vi "play_FXP_AFMss_LinearDistEst_singleAxis.vi"() -> ()   [LabVIEW 2017]
uses:
  <vilib>/rvi/interface/nirviMethod/nirviMethod.xnode
  <vilib>/rvi/errors/niLvFpgaMergeErrorWithErrorCode.vi
  <vilib>/rvi/interface/nirviReadWriteControl/nirviReadWriteControl.xnode
  <vilib>/rvi/errors/niLvFpgaAdjustHostInterfaceError.vi
  <vilib>/rvi/interface/nirviOpenFPGA/nirviOpenFPGA.xnode
  <vilib>/userdefined/High Color/nirio_resource_hc.ctl
  <vilib>/FPGAPlugInAG/Dynamic/niLvFpga_Reset_Dynamic.vi
  <vilib>/rvi/interface/Simulation/niFpgaSimulationCallBeginRW.vi
  <vilib>/FPGAPlugInAG/Dynamic/niLvFpga_Run_Dynamic.vi
  <vilib>/rvi/interface/nirviMethod/StockFPGA_InlinedMethodWaitForSingleIRQ.vi
  <vilib>/FPGAPlugInAG/Dynamic/niLvFpga_WaitOnIrq_Dynamic.vi
  <vilib>/FPGAPlugInAG/Dynamic/niLvFpga_AcknowledgeIrq_Dynamic.vi
  <vilib>/rvi/interface/nirviCloseFPGA/nirviCloseFPGA.xnode
  <vilib>/FPGAPlugInAG/Dynamic/niLvFpga_ConfigureFifo_Dynamic.vi
  <vilib>/Utility/error.llb/DialogType.ctl
  <vilib>/Analysis/Matrix/NI_Matrix.lvlib
  fpga_VIs/fpga_subVIs_ssxy/fixed-point-ss/typeDefs/FXPControlParams_distEst.ctl
  <vilib>/FPGAPlugInAG/Dynamic/niLvFpga_WriteFifo_Dynamic.vi
  <vilib>/Analysis/Matrix/Numeric/Conversions/Matrix To Array - RM.vi
  labview/utils_lib/utils.lvlib
  <vilib>/Utility/file.llb/Read Delimited Spreadsheet (DBL).vi
  fpga_interface_lib/fpga_interface.lvlib
  <vilib>/Analysis/Matrix/Numeric/Conversions/Array To Matrix - RA2.vi
  <vilib>/Utility/file.llb/Write To Spreadsheet File (DBL).vi
  fpga_interface_lib/write_FP_data_to_fpga.vi
  <vilib>/Utility/error.llb/Error Cluster From Error Code.vi
  FPGA Bitfiles/afmimagingcontro_FPGATargetSPARTA_FXPAFMssLinearDi_nzyJCj76J+U.lvbitx
  NiFpgaLv.dll
  fpga_interface_lib/acquire_FXP_18-5_FIFO_1.vi
  <vilib>/FPGAPlugInAG/Dynamic/niLvFpga_Close_Dynamic.vi
  <vilib>/FPGAPlugInAG/cRIO-9082/niLvFpga_Open_cRIO-9082.vi
  <vilib>/rvi/interface/common/dynamic/niFpgaDynamicAddResources.vi
  fpga_interface_lib/fpga_interface_types/boolean_indicators.ctl
  <vilib>/Analysis/Matrix/Datatypes/RealMatrix.ctl
panel:
  out "Array":dbl[](array[numeric])
  out "elements left":i32=1
  in  "TF Order":i32
  in  "den":T1
  in  "num":T1
  in  "Tab Control":T2(tab)
  in  "traj_path":path=path "Z:/mpc-journal/step-exps/traj_data.csv"
  in  "TsTicks":i32=1600
  in  "umax":dbl=1.0 format="%#_13g"
  in  "ymax":dbl=4.0 format="%#_13g"
  in  "Iters":i32=25
  in  "SettleTicks":i32=10
  in  "dry_run":bool=TRUE
  in  "control_data_path":path=path "Z:/afm-cs/step-exps/LinControls01.json"
  in  "outputDataPath":path=path "Z:/mpc-journal/step-exps/expOut_multiAxis_tmp.csv"
  out "ControlParams":T3={"umax"=3.0, "Ns_obs/cntrl"=0, "ref_f_VEC"=[0.0, 0.0], "du_max"=0.0, "Nbar"=0.0, "Nhyst"=0, "Nsat"=0, "Ndrift+1"=0}
  in  "ABORT":bool
  out "XY Graph":cluster{dbl[], "2D Data Out":dbl[]}[](graph)
  in  "read_file":bool=TRUE
  in  "All_matrix":T1
  in  "Ns_obs/cntrl":u8=21
  in  "yref":T1
  in  "du_max":dbl=1.0 format="%#_13g"
  out "AllMatrix":dbl[](array[numeric])
  out "ControlMatrices":T4
  out "result_data":T1
  out "boolean  indicators":T5
  out "error out":errorcluster
  out "Empty Elements Remaining":u32
  out "size(s)":i32[](array[numeric])
  out "u_k out":fxp<+/-,32,5>
  out "AllMatHS Length":i32
  # "NOTE: Ns is the number of states in the plant. The number of states in the \nobserver is Ns+1. Thus, for B, L, C, and A, we use NS+1. For K and Xss, we use Ns\nbecause the controller does not operate on the disturbance state, Xd."
  # "yk\nulin\ndu\nu_inv\nIpow\nX"
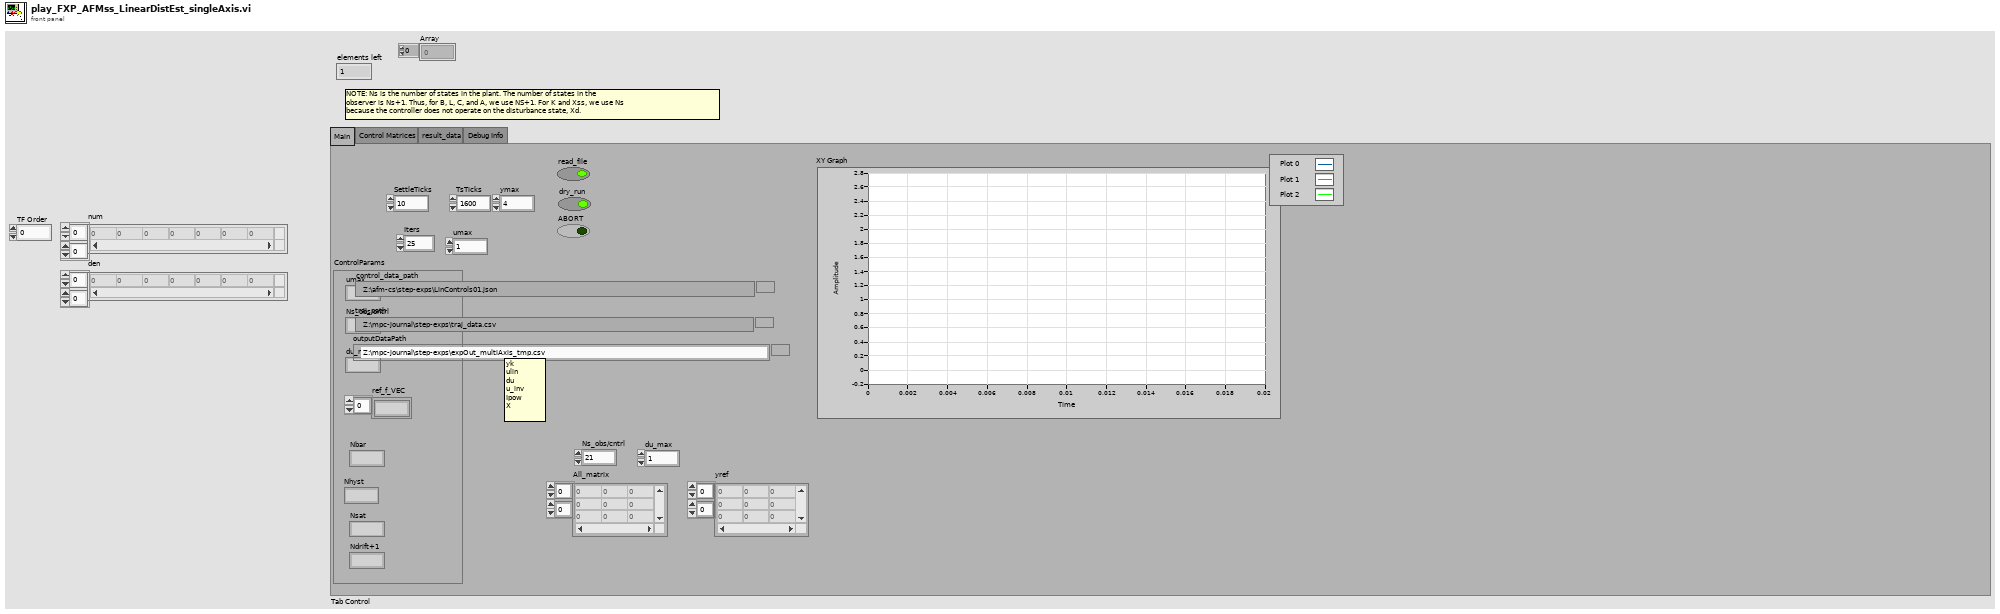
[diagram p1: front panel]
types:
  T1 = typedef "NI_Matrix.lvlib/RealMatrix.ctl" = dbl[][]
  T2 = enum32{"Main", "Control Matrices", "result_data", "Debug Info"}
  T3 = typedef "FXPControlParams_distEst.ctl" = cluster{"umax":fxp<+/-,18,5>, "Ns_obs/cntrl":u8, "ref_f_VEC":fxp<+/-,32,5>[], "du_max":fxp<+/-,18,5>, "Nbar":fxp<+/-,32,5>, "Nhyst":u8, "Nsat":u8, "Ndrift+1":u8}
  T4 = cluster{"Az":fxp<+/-,32,4>[][], "Bz":dbl[][], "Lz":dbl[][], "Kz":dbl[][], "NxNu":dbl[][]}
  T5 = typedef "fpga_interface.lvlib/boolean_indicators.ctl" = cluster{"unstable-z-traj":bool, "input fifo time-out":bool, "logging fifo timeout":bool, "scanning finished":bool, "unstable-x-traj":bool, "unstable-y-traj":bool, "ABORT":bool, "All Measurements Done":bool, "fpga_finished":bool}
  T6 = typedef "nirio_resource_hc.ctl" = tag
  T7 = typedef "ObserverMatrices.ctl" = cluster{"Az":fxp<+/-,32,4>[][], "Bz":dbl[][], "Lz":dbl[][], "Kz":dbl[][], "NxNu":dbl[][]}
  T8 = cluster{"unstable-z-traj":bool, "input fifo time-out":bool, "logging fifo timeout":bool, "scanning finished":bool, "unstable-x-traj":bool, "unstable-y-traj":bool, "ABORT":bool, "All Measurements Done":bool, "fpga_finished":bool}
  T9 = typedef "DialogType.ctl" = u16
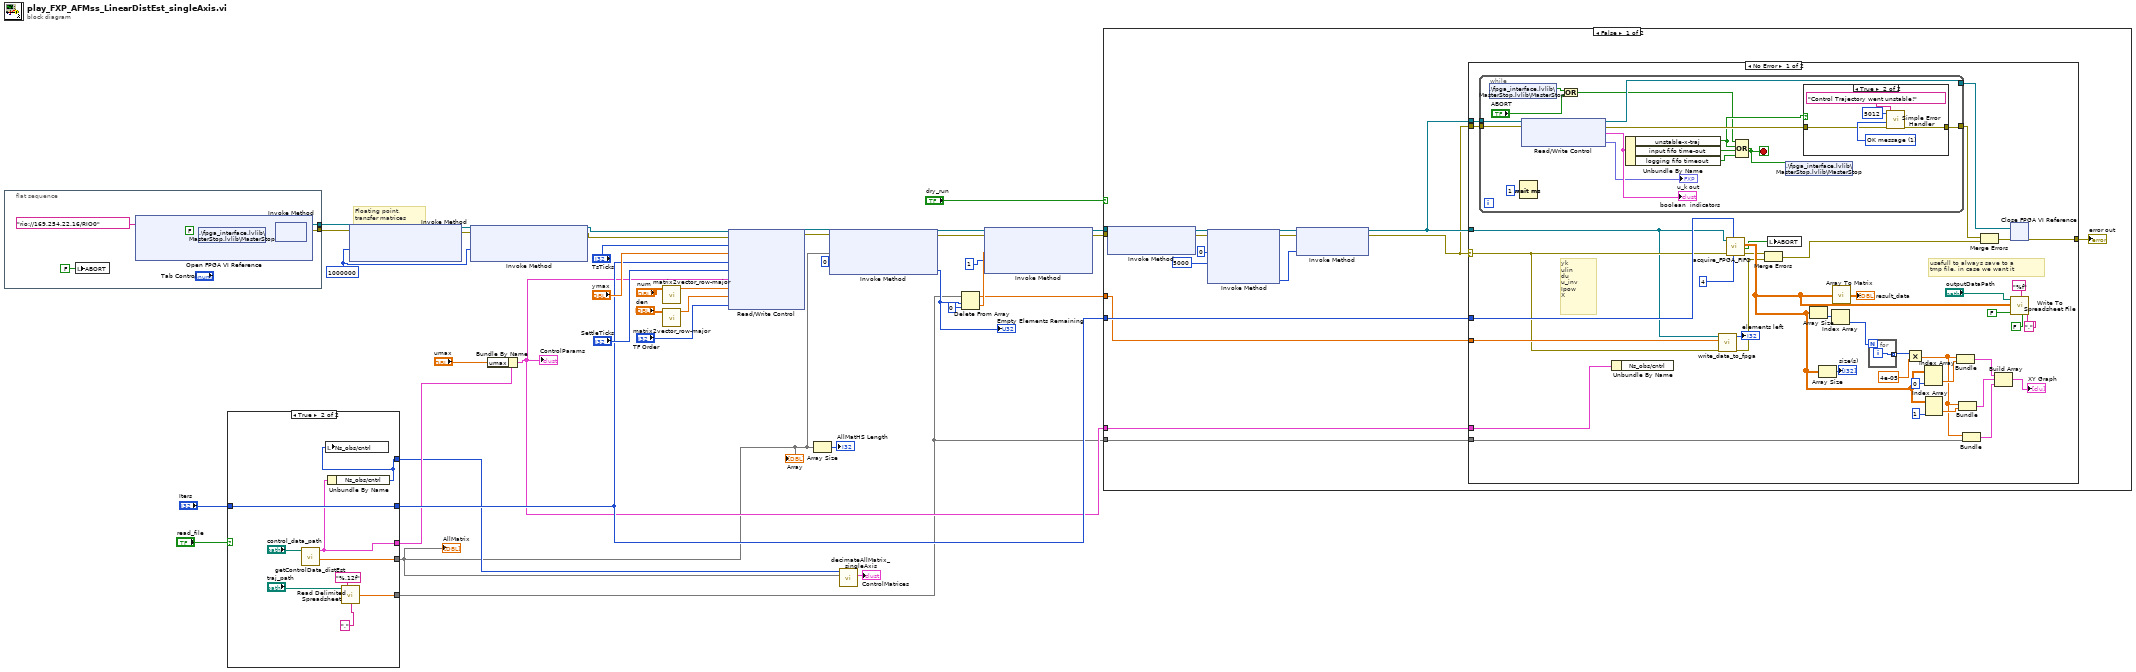
[diagram p0: block diagram]
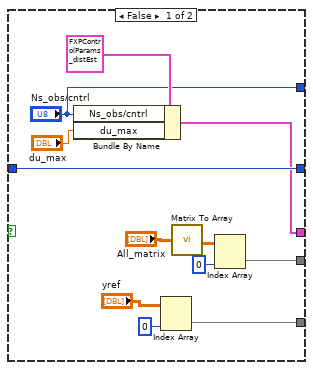
[diagram p2: hidden frame]
diagram:
  w5 = u32 1000000 ("Requested Depth")
  # "Floating point, \ntransfer matrices"
  n1 = flat-sequence {
    tunnel: [w46] -> w32
    tunnel: [w45] -> w31
    frame #0 {
      n2 = local write "ABORT"(FALSE) -> ()
      n3 = xnode "Open FPGA VI Reference"("resource name"=T6 "rio://169.254.22.16/RIO0") -> ("FPGA VI Reference Out"=w44:refnum<k20>, "error out"=w42:errorcluster)  [unwired: 1 in]
      n4 = shared-variable ".\\fpga_interface.lvlib\\MasterStop.lvlib\\MasterStop"(FALSE ("MasterStop"), error in=w42) -> (error out=w40:errorcluster)
      n5 = xnode "Invoke Method"("FPGA VI Reference In"=w44, "error in"=w40) -> ("FPGA VI Reference Out"=w46:refnum<k20>, "error out"=w45:errorcluster)
    }
  }
  n6 = case shown="True" "read_file" {
    tunnel: [w49 w61] -> w7
    tunnel: [w57 w67] -> w1
    tunnel: ["Ns_obs/cntrl" w60] -> w6
    tunnel: [w52 w64] -> w3
    tunnel: "Iters" -> [w55 w63]
    tunnel: [w55 w63] -> w8
    frame False {
      n7 = Bundle By Name(cluster=T3 {"umax"=3.0, "Ns_obs/cntrl"=0, "ref_f_VEC"=[0.0, 0.0], "du_max"=0.0, "Nbar"=0.0, "Nhyst"=0, "Nsat"=0, "Ndrift+1"=0} ("ControlParams 2"), "Ns_obs/cntrl"="Ns_obs/cntrl", "du_max"="du_max") -> (w49:T3)
      n8 = Index Array(array="yref", index (col)=0 ("disabled index (col)")) -> (element=w52:dbl[])  [unwired: 1 in]
      n9 = call-poly <vilib>:"Matrix To Array.vi"("Real Matrix"="All_matrix") -> ("Real 2D Array"=w58:dbl[][])
      n10 = Index Array(array=w58, index (col)=0 ("disabled index (col)")) -> (element=w57:dbl[])  [unwired: 1 in]
    }
    frame True {
      n11 = call "getControlData_distEst.vi"("system data path"="control_data_path") -> ("AllMatrix"=w67:dbl[], "ControlParams"=w61:T3)  [unwired: 7 in, 2 out]
      n12 = Unbundle By Name(w61) -> ("Ns_obs/cntrl"=w60:u8)
      n13 = local write "Ns_obs/cntrl"(w60) -> ()
      n14 = call-poly <vilib>:"Read Delimited Spreadsheet.vi"("file path (dialog if empty)"="traj_path", "format (%.3f)"="%.12f", "delimiter (\\t)"="," ("format (%.3f)")) -> ("first row"=w64:dbl[])  [unwired: 7 in, 5 out]
    }
  }
  "AllMatrix" <- w1
  "Array" <- w1
  n15 = xnode "Invoke Method"("FPGA VI Reference In"=w32, "error in"=w31, "Requested Depth"=w5) -> ("FPGA VI Reference Out"=w30:refnum<k20>, "error out"=w29:errorcluster)  [unwired: 1 out]
  n16 = xnode "Invoke Method"("FPGA VI Reference In"=w30, "error in"=w29, "Requested Depth"=w5) -> ("FPGA VI Reference Out"=w27:refnum<k20>, "error out"=w28:errorcluster)  [unwired: 1 out]
  n17 = Bundle By Name(cluster=w7, "umax"="umax") -> (w4:T3)
  "ControlParams" <- w4
  n18 = call "matrix2vector_row-major.vi"("Matrix"="num") -> ("vector"=w21:dbl[])  [unwired: 10 in]
  n19 = call "matrix2vector_row-major.vi"("Matrix"="den") -> ("vector"=w20:dbl[])  [unwired: 10 in]
  n20 = xnode "Read/Write Control"("FPGA VI Reference In"=w27, "error in"=w28, "TsTicks"="TsTicks", "ymax"="ymax", "iters"=w8, "Settle Ticks"="SettleTicks", "ControlParamsMpc"=w4, "Num"=w21, "Den"=w20, "TF Order"="TF Order") -> ("FPGA VI Reference Out"=w36:refnum<k20>, "error out"=w35:errorcluster)
  n21 = Array Size(array=w1) -> (size(s)=→"AllMatHS Length":i32)
  n22 = xnode "Invoke Method"("FPGA VI Reference In"=w36, "error in"=w35, "Data"=w1, "Timeout (ms)"=0) -> ("FPGA VI Reference Out"=w14:refnum<k20>, "error out"=w13:errorcluster, "Empty Elements Remaining"=w12:u32)
  "Empty Elements Remaining" <- w12
  n23 = call "decimateAllMatrix_singleAxis.vi"("AllMatrix"=w1, "NS_obs/cntrl"=w6) -> ("ControlMatrices"=→"ControlMatrices":T7)  [unwired: 8 in, 1 out]
  n24 = Delete From Array(array=w3, length=w12, index=0) -> (deleted portion=w18:dbl[], array with subset deleted=w10:dbl[])
  n25 = xnode "Invoke Method"("FPGA VI Reference In"=w14, "error in"=w13, "Data"=w18, "Timeout (ms)"=1) -> ("FPGA VI Reference Out"=w16:refnum<k20>, "error out"=w15:errorcluster)  [unwired: 1 out]
  n26 = case shown="False" "dry_run" {
    tunnel: w16 -> [w84 _]
    tunnel: w15 -> [w83 _]
    tunnel: w8 -> [w74 _]
    tunnel: w10 -> [w73 _]
    tunnel: w3 -> [w72 _]
    tunnel: w4 -> [w71 _]
    frame False {
      n27 = xnode "Invoke Method"("FPGA VI Reference In"=w84, "error in"=w83) -> ("FPGA VI Reference Out"=w77:refnum<k20>, "error out"=w78:errorcluster)  [unwired: 1 in]
      n28 = xnode "Invoke Method"("FPGA VI Reference In"=w77, "error in"=w78, "IRQ Number(s)"=0, "Timeout (ms)"=5000) -> ("FPGA VI Reference Out"=w81:refnum<k20>, "error out"=w82:errorcluster, "IRQ(s) Asserted"=w80:i32)  [unwired: 1 out]
      n29 = xnode "Invoke Method"("FPGA VI Reference In"=w81, "error in"=w82, "IRQ Number(s)"=w80) -> ("FPGA VI Reference Out"=w70:refnum<k20>, "error out"=w69:errorcluster)
      n30 = case shown="No Error" w69 {
        selector: w69 -> [w100 w146]
        tunnel: [w122 w146] -> w75
        tunnel: w70 -> [w121 _]
        tunnel: w69 -> [w120 _]
        tunnel: w74 -> [w117 _]
        tunnel: w70 -> [w90 _]
        tunnel: w73 -> [w101 _]
        tunnel: w72 -> [w94 _]
        tunnel: w71 -> [w91 _]
        frame No Error {
          # "yk\nulin\ndu\nu_inv\nIpow\nX"
          # "usefull to always save to a \ntmp file, in case we want it"
          n31 = while {
            tunnel: w121 -> [w138]
            tunnel: w120 -> [w137]
            tunnel: [w135] -> w119
            tunnel: [w134] -> w118
            stop <- w125 stop-if-true
            n32 = shared-variable ".\\fpga_interface.lvlib\\MasterStop.lvlib\\MasterStop"() -> (w126:bool)  [unwired: 1 in, 1 out]
            n33 = Wait (ms)(milliseconds to wait=u32 1) -> ()  [unwired: 1 out]
            n34 = xnode "Read/Write Control"("FPGA VI Reference In"=w138, "error in"=w137) -> ("FPGA VI Reference Out"=w134:refnum<k20>, "error out"=w136:errorcluster, "boolean indicators"=w133:T8, "u_k"=→"u_k out":fxp<+/-,32,5>)
            "boolean  indicators" <- w133
            n35 = Or(x=w126, y="ABORT") -> (x .or. y?=w128:bool)
            n36 = Unbundle By Name(w133) -> ("unstable-x-traj"=w131:bool, "input fifo time-out"=w132:bool, "logging fifo timeout"=w130:bool)
            n37 = Compound Arithmetic op=OR(w128, w131, w132, w130) -> (w125:bool)
            n38 = shared-variable ".\\fpga_interface.lvlib\\MasterStop.lvlib\\MasterStop"(w125) -> ()  [unwired: 1 in, 1 out]
            n39 = case shown="True" w131 {
              tunnel: w136 -> [w140 w142]
              tunnel: [w140 w141] -> w135
              frame False {
              }
              frame True {
                w145 = T9 1 items=["no dialog", "OK message", "continue or stop message", "OK message + warnings", "continue/stop + warnings"] ("type of dialog (OK msg:1)")
                n40 = call <vilib>:"Simple Error Handler.vi"("error code (no error:0)"=5012, "error source (\" \")"="Control Trajectory went unstable!" ("error source (\" \")"), "type of dialog (OK msg:1)"=w145, "error in (no error)"=w142) -> ("error out"=w141:errorcluster)  [unwired: 1 in, 4 out]
              }
            }
          }
          n41 = Unbundle By Name(w91) -> ()  [unwired: 1 out]
          n42 = call-poly "write_data_to_fpga.vi"("error in"=w100, "all rows"=w101, "FPGA Interface"=w90) -> ("error out"=w97:errorcluster, "elements left"=→"elements left":i32)  [unwired: 7 in]
          n43 = call-poly "acquire_FPGA_FIFO.vi"("numChannels"=u8 4 ("y"), "Iters"=w117, "error in"=w100, "FPGA Interface"=w90) -> ("error out"=w99:errorcluster, "finished"=w85:bool, "2D Data Out"=w115:dbl[][])  [unwired: 2 in, 3 out]
          n44 = Merge Errors(w99, w97) -> (w98:errorcluster)
          n45 = local write "ABORT"(w85) -> ()
          n46 = Array Size(array=w115) -> (size(s)=w111:i32[])
          n47 = Array Size(array=w115) -> (size(s)=→"size(s)":i32[])
          n48 = Index Array(array=w111) -> (element=w110:i32)  [unwired: 1 in]
          n49 = call-poly <vilib>:"Array To Matrix.vi"("Real 2D Array"=w115) -> ("Real Matrix"=→"result_data":T1)
          n50 = for {
            N: w110 -> [_]
            tunnel: [w124] -> w109 mode=indexing
            i -> [w124]
          }
          n51 = Multiply(x=w109, y=4e-05) -> (x*y=w95:dbl[])
          n52 = Index Array(array=w115, index (col)=0 ("disabled index (col)")) -> (element=w107:dbl[])  [unwired: 1 in]
          n53 = Index Array(array=w115, index (col)=1 ("index (row)")) -> (element=w106:dbl[])  [unwired: 1 in]
          n54 = Bundle(w95, "2D Data Out"=w107) -> (w88:cluster{dbl[], "2D Data Out":dbl[]})  [unwired: 1 in]
          n55 = Bundle(w95, "2D Data Out"=w106) -> (w87:cluster{dbl[], "2D Data Out":dbl[]})  [unwired: 1 in]
          n56 = Bundle(w95, "first row"=w94) -> (w86:cluster{dbl[], "first row":dbl[]})  [unwired: 1 in]
          n57 = Merge Errors(w119, w98) -> (w123:errorcluster)
          n58 = Build Array(w88, w87, w86) -> (→"XY Graph":cluster{dbl[], "first row":dbl[]}[])
          n59 = xnode "Close FPGA VI Reference"("FPGA VI Reference In"=w118, "error in"=w123) -> ("error out"=w122:errorcluster)
          n60 = call-poly <vilib>:"Write To Spreadsheet File.vi"("delimiter (\\t)"=",", "transpose? (no:F)"=FALSE, "format (%.3f)"="%f", "append to file? (new file:F)"=FALSE, "2D data"=w115, "file path (dialog if empty)"="outputDataPath") -> ()  [unwired: 2 in, 1 out]
        }
        frame Error {
        }
      }
      "error out" <- w75
    }
    frame True {
    }
  }
